vi "Set Gain and Phase.vi"(8 "error in (no error)":errorcluster, 10 "Gain and Phase":T1 {"Phase SD" format="%.1f"; "Phase" format="%.1f"; "Gain SD" format="%.2f"; "Gain" format="%.2f"}, 11 "Sinusoidal Fit in":refnum<class "Sinusoidal Fit.lvclass">) -> (0 "error out":errorcluster, 3 "Sinusoidal Fit out":refnum<class "Sinusoidal Fit.lvclass">)   [LabVIEW 2013, in "Sinusoidal Fit.lvclass"]
uses:
  Sinusoidal Fit.lvclass
  gain and phase/Typedef - Gain and Phase.ctl
  Sinusoidal Fit.lvclass/Sinusoidal Fit.ctl
panel:
  # "Gain:"
  # "+/-"
  # "Phase:"
  # "+/-"
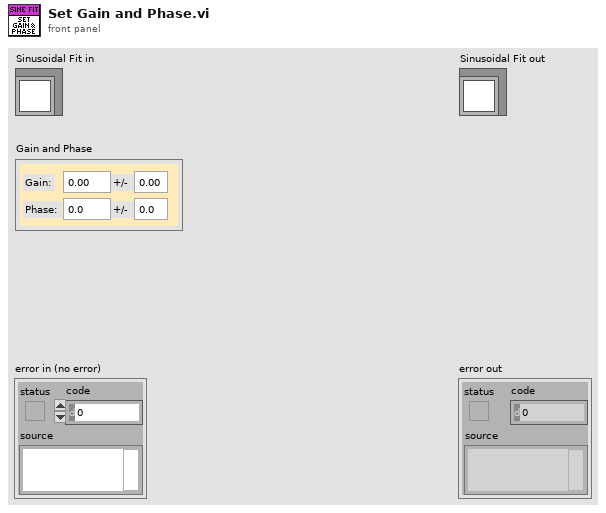
[diagram p1: front panel]
types:
  T1 = typedef "Typedef - Gain and Phase.ctl" = cluster{"Gain":dbl, "Gain SD":dbl, "Phase":dbl, "Phase SD":dbl}
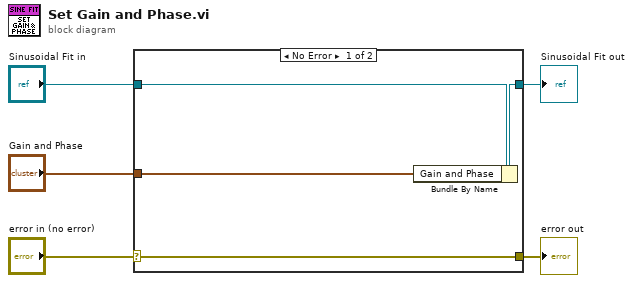
[diagram p0: block diagram]
diagram:
  n1 = case shown="No Error" "error in (no error)" {
    selector: "error in (no error)" -> [w9 w10]
    tunnel: [w9 w10] -> w4
    tunnel: [w7 w11] -> w2
    tunnel: "Sinusoidal Fit in" -> [w8 w11]
    tunnel: "Gain and Phase" -> [w6 _]
    frame No Error {
      n2 = Bundle By Name(cluster=w8, "Gain and Phase"=w6) -> (w7:refnum<class "Sinusoidal Fit.lvclass">)
    }
    frame Error {
    }
  }
  "error out" <- w4
  "Sinusoidal Fit out" <- w2
